vi "SSI_check packet.vi"(2 "input":i32, 3 "input loss":i32) -> (0 "array":i32[](array[numeric]), 1 "loss count":i32=-1)   [LabVIEW 2011]
panel:
  out "packcnt":i32
  out "buffer cnt":i32
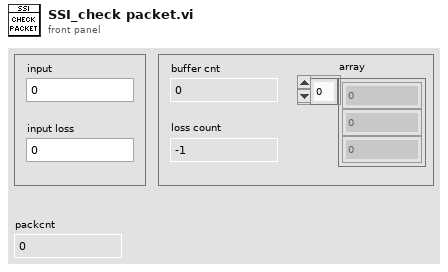
[diagram p1: front panel]
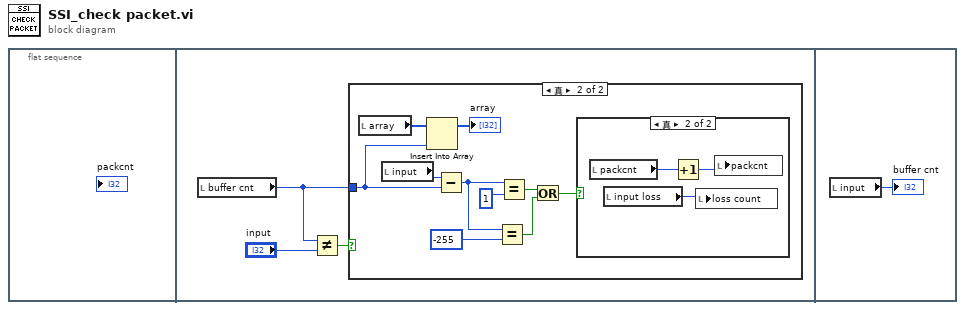
[diagram p0: block diagram]
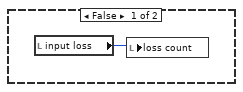
[diagram p2: hidden frame]
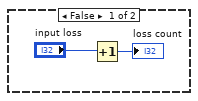
[diagram p3: hidden frame]
diagram:
  n1 = flat-sequence {
    frame #0 {
    }
    frame #1 {
      n2 = local read "buffer cnt"() -> (w2:i32)
      n3 = Not Equal?(x=w2, y="input") -> (x != y?=w3:bool)
      n4 = case shown="真" w3 {
        tunnel: w2 -> [_ w6]
        frame False {
          n5 = local read "input loss"() -> (w4:i32)
          n6 = local write "loss count"(w4) -> ()
        }
        frame True {
          n7 = local read "array"() -> (w7:i32[])
          n8 = local read "input"() -> (w14:i32)
          n9 = Insert Into Array(array=w7, new element=w6) -> (→"array":i32[])  [unwired: 1 in]
          n10 = Subtract(x=w14, y=w6) -> (x-y=w12:i32)
          n11 = Equal?(x=w12, y=-255) -> (x = y?=w9:bool)
          n12 = Equal?(x=w12, y=1) -> (x = y?=w10:bool)
          n13 = Or(x=w10, y=w9) -> (x .or. y?=w8:bool)
          n14 = case shown="真" w8 {
            frame False {
              n15 = Increment(x="input loss") -> (x+1=→"loss count":i32)
            }
            frame True {
              n16 = local read "packcnt"() -> (w18:i32)
              n17 = local read "input loss"() -> (w19:i32)
              n18 = Increment(x=w18) -> (x+1=w17:i32)
              n19 = local write "loss count"(w19) -> ()
              n20 = local write "packcnt"(w17) -> ()
            }
          }
        }
      }
    }
    frame #2 {
      n21 = local read "input"() -> (→"buffer cnt":i32)
    }
  }
